vi "_getChannelLength.vi"(4 "error in (no error)":errorcluster, 7 "channel refnum in":refnum<k20>) -> (0 "error out":errorcluster, 2 "channel length":i32, 3 "channel refnum out":refnum<k20>)   [LabVIEW 2020]
uses:
  __loadPropRefList.vi
  __loadPropInt32.vi
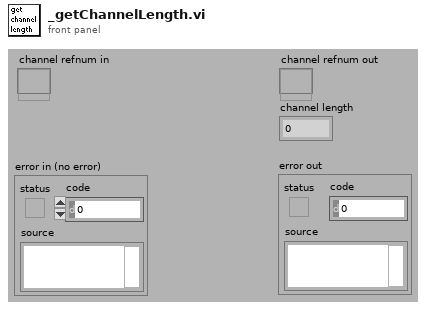
[diagram p1: front panel]
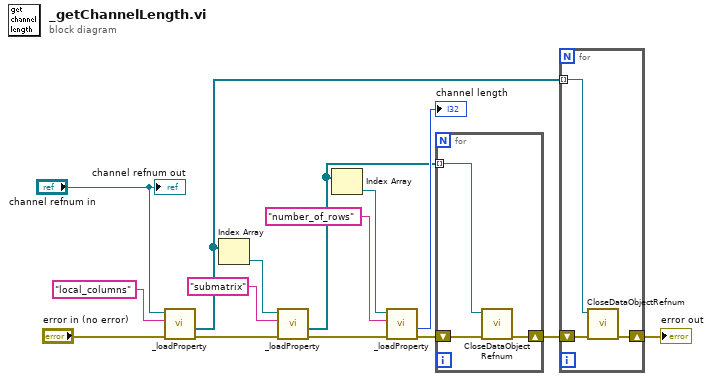
[diagram p0: block diagram]
diagram:
  n1 = call-poly "_loadProperty.vi"("error in (no error)"="error in (no error)", "Property name"="local_columns", "storage refnum"="channel refnum in") -> ("error out"=w13:errorcluster, "Value"=w3:refnum<k20>[])  [unwired: 6 in, 1 out]
  n2 = Index Array(array=w3) -> (element=w8:refnum<k20>)  [unwired: 1 in]
  n3 = call-poly "_loadProperty.vi"("error in (no error)"=w13, "Property name"="submatrix", "storage refnum"=w8) -> ("error out"=w14:errorcluster, "Value"=w5:refnum<k20>[])  [unwired: 6 in, 1 out]
  n4 = Index Array(array=w5) -> (element=w10:refnum<k20>)  [unwired: 1 in]
  n5 = call-poly "_loadProperty.vi"("error in (no error)"=w14, "Property name"="number_of_rows", "storage refnum"=w10) -> ("error out"=w4:errorcluster, "Value"=→"channel length":i32)  [unwired: 6 in, 1 out]
  n6 = for {
    tunnel: w5 -> [w18] mode=indexing
    shift-right: [w16] -> w2
    shift-left: w4 -> [w17]
    n7 = call "CloseDataObjectRefnum.vi"("error in (no error)"=w17, "storage refnum"=w18) -> ("error out"=w16:errorcluster)  [unwired: 9 in]
  }
  n8 = for {
    tunnel: w3 -> [w21] mode=indexing
    shift-right: [w19] -> w1
    shift-left: w2 -> [w20]
    n9 = call "CloseDataObjectRefnum.vi"("error in (no error)"=w20, "storage refnum"=w21) -> ("error out"=w19:errorcluster)  [unwired: 9 in]
  }
  "error out" <- w1
  "channel refnum out" <- "channel refnum in"
